vi "FetchWeek.vi"(7 "WeeklyRootPath":path=path "C:/data/comics/weeklies", 9 "Save to disk?":bool=TRUE, 11 "time stamp":timestamp) -> (0 "error out":errorcluster, 1 "Retries":i32, 3 "body":string)   [LabVIEW 2022 SP3]
uses:
  TypeDefs/LoCG_RootURL.ctl
  <vilib>/Utility/file.llb/Write Delimited Spreadsheet (string).vi
panel:
  out "Weekly URL":string
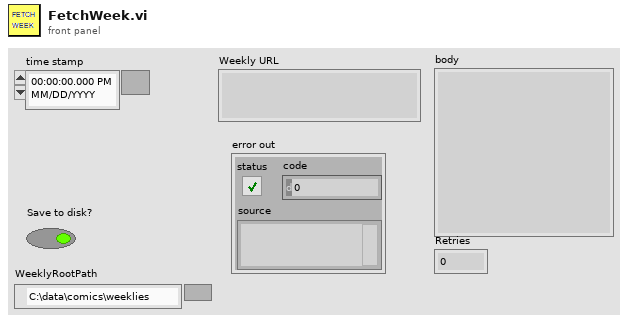
[diagram p1: front panel]
types:
  T1 = typedef "LoCG_RootURL.ctl" = string
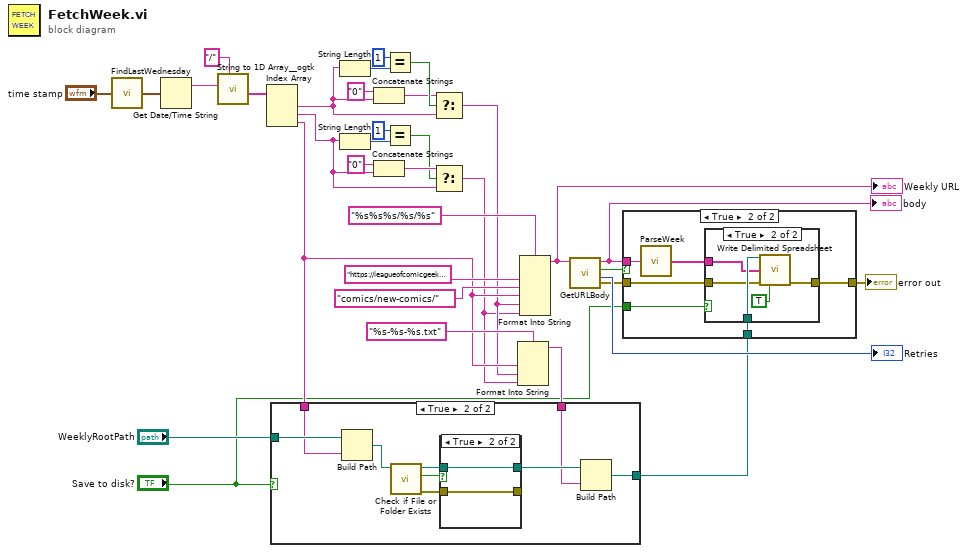
[diagram p0: block diagram]
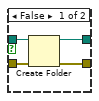
[diagram p5: hidden frame]
diagram:
  n1 = call "FindLastWednesday.vi"("current time"="time stamp") -> ("Most Recent Wednesday"=w15:timestamp)
  n2 = Get Date/Time String(seconds (now)=w15) -> (date string=w33:string)  [unwired: 2 in, 1 out]
  n3 = call <userlib>:"String to 1D Array__ogtk.vi"("delimiter (Tab)"="/", "string"=w33) -> ("Array of Strings"=w30:string[])  [unwired: 9 in]
  n4 = Index Array(array=w30) -> (element #1=w26:string, element #2=w20:string, element #3=w9:string)  [unwired: 3 in]
  n5 = String Length(string=w26) -> (length=w32:i32)
  n6 = String Length(string=w20) -> (length=w21:i32)
  n7 = Concatenate Strings("0" ("string"), w26) -> (w27:string)
  n8 = Concatenate Strings("0" ("string"), w20) -> (w25:string)
  n9 = Equal?(x=1, y=w32) -> (x = y?=w29:bool)
  n10 = Equal?(x=1, y=w21) -> (x = y?=w23:bool)
  n11 = Select(t=w27, s=w29, f=w26) -> (s? t:f=w8:string)
  n12 = Select(t=w25, s=w23, f=w20) -> (s? t:f=w7:string)
  n13 = Format Into String(format string="%s-%s-%s.txt", w9, w8, w7) -> (resulting string=w11:string)  [unwired: 2 in, 1 out]
  n14 = case shown="True" "Save to disk?" {
    tunnel: w11 -> [_ w39]
    tunnel: "WeeklyRootPath" -> [_ w38]
    tunnel: w9 -> [_ w36]
    tunnel: [_ w35] -> w5
    frame False {
    }
    frame True {
      n15 = Build Path(base path=w38, name or relative path=w36) -> (appended path=w41:path)
      n16 = call <vilib>:"Check if File or Folder Exists.vi"("path"=w41) -> ("error out"=w37:errorcluster, "file or folder exists?"=w42:bool, "dup path"=w43:path)  [unwired: 8 in]
      n17 = case shown="True" w42 {
        tunnel: [w47 w49] -> w40
        tunnel: [w46 w48] -> _
        tunnel: w37 -> [w45 w48]
        tunnel: w43 -> [w44 w49]
        frame False {
          n18 = Create Folder(path (use dialog)=w44, error in=w45) -> (created path=w47:path, error out=w46:errorcluster)  [unwired: 1 in, 1 out]
        }
        frame True {
        }
      }
      n19 = Build Path(base path=w40, name or relative path=w39) -> (appended path=w35:path)
    }
  }
  n20 = Format Into String(format string="%s%s%s/%s/%s", T1 "https://leagueofcomicgeeks.com/" ("LoCG Root Path"), "comics/new-comics/", w9, w8, w7) -> (resulting string=w14:string)  [unwired: 2 in, 1 out]
  "Weekly URL" <- w14
  n21 = call "GetURLBody.vi"("URL"=w14) -> ("error out"=w4:errorcluster, "Retries"=→"Retries":i32, "Success?"=w2:bool, "body"=w6:string)  [unwired: 7 in]
  "body" <- w6
  n22 = case shown="True" w2 {
    tunnel: w6 -> [_ w56]
    tunnel: w5 -> [_ w55]
    tunnel: w4 -> [w50 w54]
    tunnel: [w50 w52] -> w3
    tunnel: "Save to disk?" -> [_ w51]
    frame False {
    }
    frame True {
      n23 = call "ParseWeek.vi"("HTML  Body"=w56) -> ("ComicURLs"=w53:string[])
      n24 = case shown="True" w51 {
        tunnel: w55 -> [_ w62]
        tunnel: w54 -> [w57 w61]
        tunnel: w53 -> [_ w60]
        tunnel: [w57 w59] -> w52
        frame False {
        }
        frame True {
          n25 = call-poly <vilib>:"Write Delimited Spreadsheet.vi"("file path (dialog if empty)"=w62, "1D data"=w60, "error in (no error)"=w61, "transpose? (no:F)"=TRUE) -> ("error out"=w59:errorcluster)  [unwired: 10 in, 1 out]
        }
      }
    }
  }
  "error out" <- w3
